vi "Destroy.vi"(8 "error in (no error)":errorcluster, 11 "selection_dropdown in":refnum<class "selection_dropdown.lvclass">) -> (0 "error out":errorcluster, 3 "selection_dropdown out":refnum<class "selection_dropdown.lvclass">)   [LabVIEW 2024, in "selection_dropdown.lvclass"]
uses:
  selection_dropdown.lvclass
  selection_dropdown.lvclass/selection_dropdown.ctl
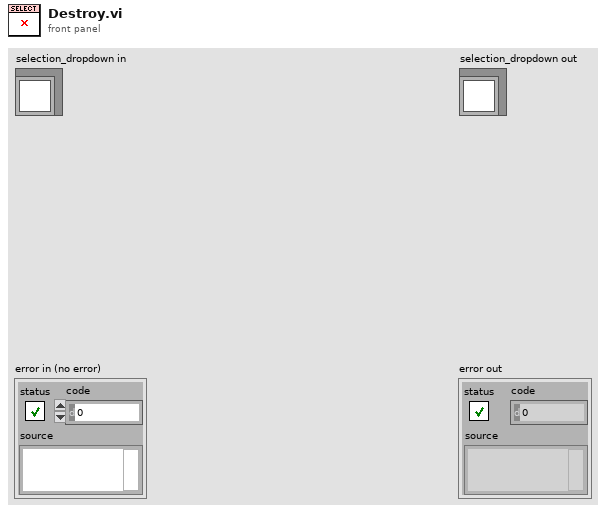
[diagram p1: front panel]
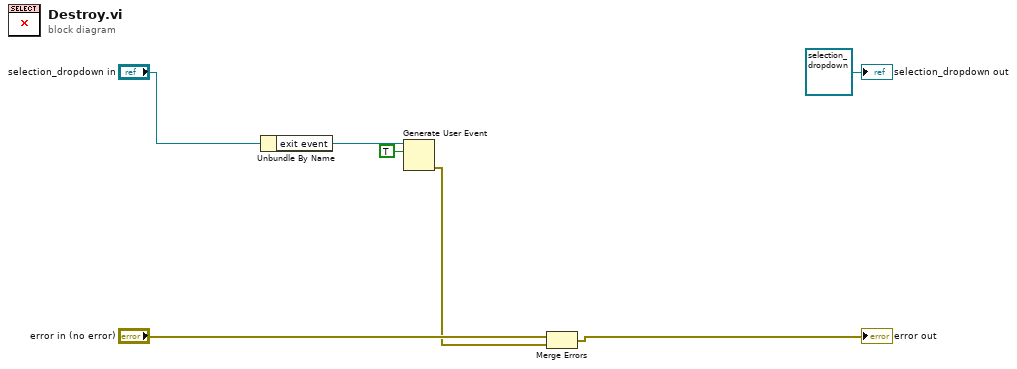
[diagram p0: block diagram]
diagram:
  n1 = Unbundle By Name("selection_dropdown in") -> ("exit event"=w6:refnum<user-event>)
  n2 = Generate User Event(user event=w6, event data cluster=TRUE ("event data")) -> (error out=w2:errorcluster)  [unwired: 2 in, 1 out]
  n3 = Merge Errors("error in (no error)", w2) -> (→"error out":errorcluster)
  "selection_dropdown out" <- refnum<class "selection_dropdown.lvclass"> refnum ("selection_dropdown out")
